vi "cmbBox Change List and Set Value.vi"(8 "error in (no error)":errorcluster, 10 "Strings []":string[](array[string]), 11 "cmbBox":refnum<vi>) -> (0 "error out":errorcluster, 3 "cmbBox(dup)":refnum<vi>)   [LabVIEW 2017, in "csm-ui-support.lvlib"]
uses:
  csm-ui-support.lvlib
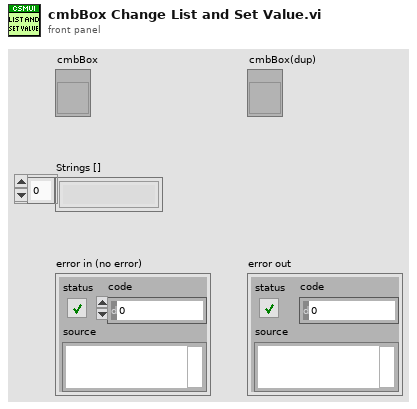
[diagram p1: front panel]
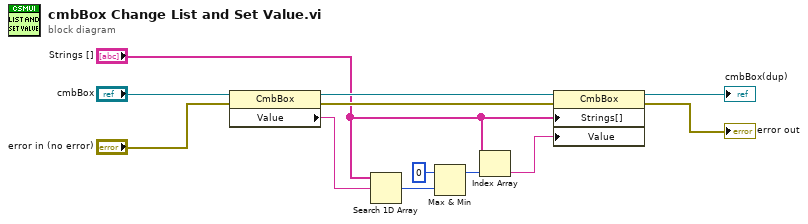
[diagram p0: block diagram]
diagram:
  n1 = property on="Property Node" class="CmbBox"(reference="cmbBox", error in="error in (no error)") -> (reference out=w10:refnum<vi>, error out=w11:errorcluster, "Value"=w12:string)
  n2 = Search 1D Array(1D array="Strings []", element=w12) -> (index of element=w7:i32)  [unwired: 1 in]
  n3 = Max & Min(x=0, y=w7) -> (max(x,y)=w4:i32)  [unwired: 1 out]
  n4 = Index Array(array="Strings []", index=w4) -> (element=w6:string)
  n5 = property on="Property Node" class="CmbBox"(reference=w10, error in=w11, "Strings[]"="Strings []", "Value"=w6) -> (reference out=→"cmbBox(dup)":refnum<vi>, error out=→"error out":errorcluster)
